vi "xmlStringWriteInt.vi"(4 "Value":i32) -> (1 "String":string)   [LabVIEW 2012]
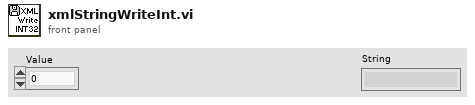
[diagram p1: front panel]
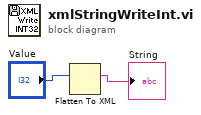
[diagram p0: block diagram]
diagram:
  n1 = Flatten To XML(anything="Value") -> (xml string=→"String":string)
